vi "Noyito10ChannelADC_CalculateMeanAllChannels.vi"(10 "ADC Counts":T2(array[cluster]), 11 "ADC Voltages":T1(array[cluster])) -> (2 "ADC Counts - Mean Values":T3, 3 "ADC Voltages - Mean Values":T3)   [LabVIEW 2020]
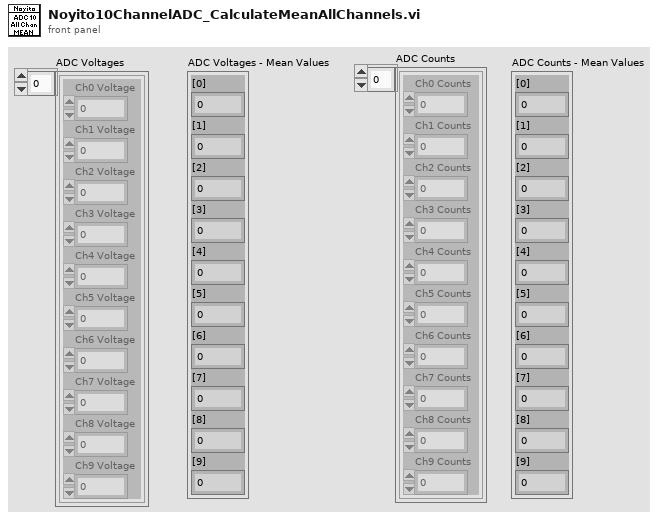
[diagram p1: front panel]
types:
  T1 = cluster{"Ch0 Voltage":dbl, "Ch1 Voltage":dbl, "Ch2 Voltage":dbl, "Ch3 Voltage":dbl, "Ch4 Voltage":dbl, "Ch5 Voltage":dbl, "Ch6 Voltage":dbl, "Ch7 Voltage":dbl, "Ch8 Voltage":dbl, "Ch9 Voltage":dbl}[]
  T2 = cluster{"Ch0 Counts":u16, "Ch1 Counts":u16, "Ch2 Counts":u16, "Ch3 Counts":u16, "Ch4 Counts":u16, "Ch5 Counts":u16, "Ch6 Counts":u16, "Ch7 Counts":u16, "Ch8 Counts":u16, "Ch9 Counts":u16}[]
  T3 = cluster{"[0]":dbl, "[1]":dbl, "[2]":dbl, "[3]":dbl, "[4]":dbl, "[5]":dbl, "[6]":dbl, "[7]":dbl, "[8]":dbl, "[9]":dbl}
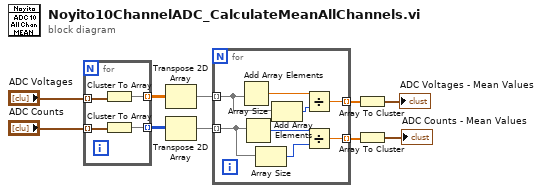
[diagram p0: block diagram]
diagram:
  n1 = for {
    tunnel: "ADC Voltages" -> [w14] mode=indexing
    tunnel: "ADC Counts" -> [w13] mode=indexing
    tunnel: [w12] -> w3 mode=indexing
    tunnel: [w11] -> w4 mode=indexing
    n2 = Cluster To Array(cluster=w14) -> (array=w12:dbl[])
    n3 = Cluster To Array(cluster=w13) -> (array=w11:u16[])
  }
  n4 = Transpose 2D Array(2D array=w3) -> (transposed array=w5:dbl[][])
  n5 = Transpose 2D Array(2D array=w4) -> (transposed array=w6:u16[][])
  n6 = for {
    tunnel: w5 -> [w18] mode=indexing
    tunnel: w6 -> [w17] mode=indexing
    tunnel: [w16] -> w7 mode=indexing
    tunnel: [w15] -> w8 mode=indexing
    n7 = Add Array Elements(numeric array=w18) -> (sum=w22:dbl)
    n8 = Add Array Elements(numeric array=w17) -> (sum=w21:u16)
    n9 = Array Size(array=w17) -> (size(s)=w20:i32)
    n10 = Array Size(array=w18) -> (size(s)=w19:i32)
    n11 = Divide(x=w22, y=w19) -> (x/y=w16:dbl)
    n12 = Divide(x=w21, y=w20) -> (x/y=w15:dbl)
  }
  n13 = Array To Cluster(array=w7) -> (cluster=→"ADC Voltages - Mean Values":T3)
  n14 = Array To Cluster(array=w8) -> (cluster=→"ADC Counts - Mean Values":T3)
